vi "bus_button.vi"(3 "Container State":T3 caption="컨테이너 상태", 4 "Previous State":variant caption="이전 상태", 5 "Previous Version":T2 caption="이전 버전") -> (2 "Current State":T1 caption="현재 상태")   [LabVIEW 2014, in "bus_button.xctl"]
uses:
  bus_button.xctl
  Normal.ctl
  <vilib>/_xctls/Container State.ctl
  <vilib>/_xctls/Version.ctl
  <vilib>/_xctls/XControlSupport.lvlib
panel:
  in  "Default Indicator State":T1 caption="기본 인디케이터 상태"
  in  "Default Control State":T1 caption="기본 컨트롤 상태"
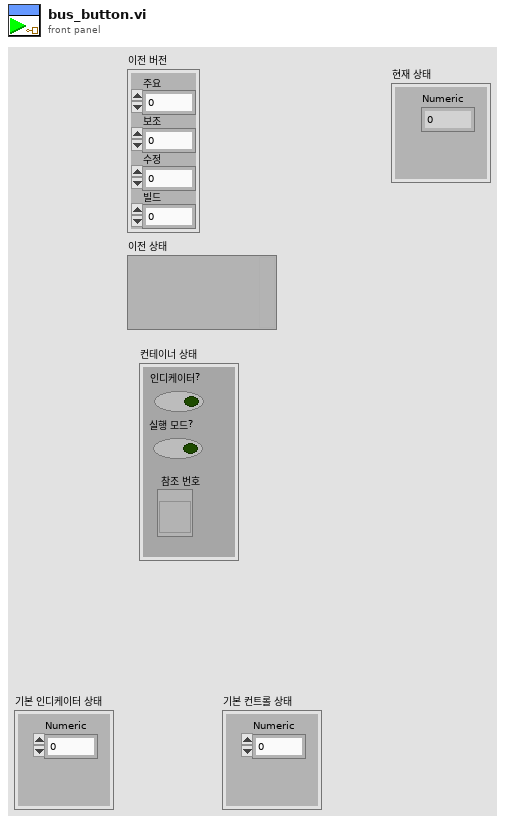
[diagram p1: front panel]
types:
  T1 = typedef "bus_button.xctl/Normal.ctl" = cluster{"Numeric":dbl}
  T2 = typedef "XControlSupport.lvlib/Version.ctl" = cluster{"Major":u16, "Minor":u16, "Fix":u16, "Build":u16}
  T3 = typedef "XControlSupport.lvlib/Container State.ctl" = cluster{"Indicator?":bool, "Run Mode?":bool, " Refnum":refnum<vi>}
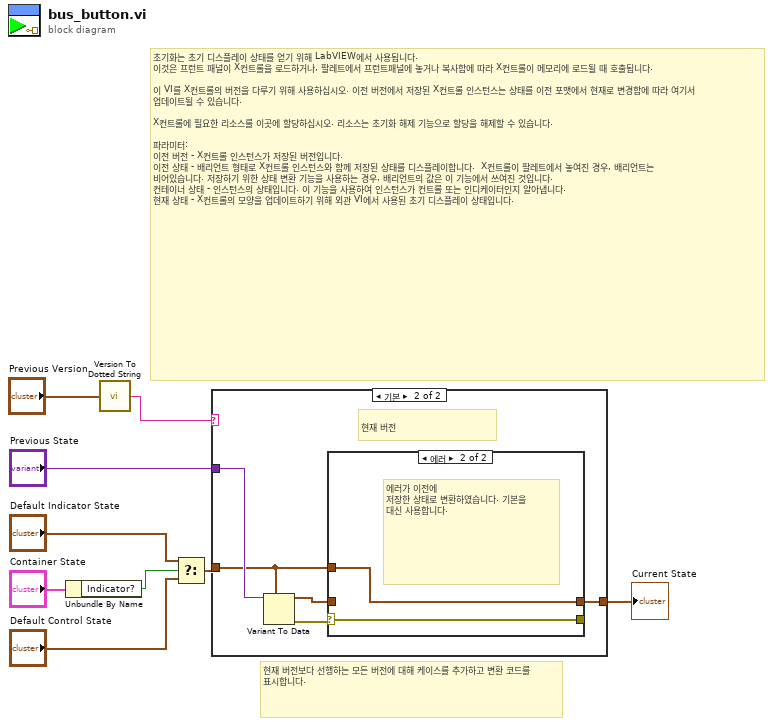
[diagram p0: block diagram]
diagram:
  # "현재 버전보다 선행하는 모든 버전에 대해 케이스를 추가하고 변환 코드를 표시합니다."
  # "초기화는 초기 디스플레이 상태를 얻기 위해 LabVIEW에서 사용됩니다.\n이것은 프런트 패널이 X컨트롤을 로드하거나, 팔레트에서 프런트패널에 놓거나 복사함에 따라 X컨트롤이 메모리에 로드될 때 호출됩니다.\n\n이 VI를 X컨트롤의 버전을 다루기 위해 사용하십시오. 이전 버전에서 저장된 X컨트롤 인스턴스는 상태를 이전 포맷에서 현재로 변경함에 따라 여기서 업데이트될 수 있습니다.\n\nX컨트롤에 필요한 리소스를 이곳에 할당하십시오. 리소스는 초기화 해제 기능으로 할당을 해제할 수 있습니다.\n\n파라미터:\n이전 버전 - X컨트롤 인스턴스가 저장된 버전입니다.\n이전 상태 - 배리언트 형태로 X컨트롤 인스턴스와 함께 저장된 상태를 디스플레이합니다.  X컨트롤이 팔레트에서 놓여진 경우, 배리언트는 비어있습니다. 저장하기 위한 상태 변환 기능을 사용하는 경우, 배리언트의 값은 이 기능에서 쓰여진 것입니다. \n컨테이너 상태 - 인스턴스의 상태입니다. 이 기능을 사용하여 인스턴스가 컨트롤 또는 인디케이터인지 알아냅니다.\n현재 상태 - X컨트롤의 모양을 업데이트하기 위해 외관 VI에서 사용된 초기 디스플레이 상태입니다."
  n1 = Unbundle By Name("Container State") -> ("Indicator?"=w4:bool)
  n2 = call <vilib>:"Version To Dotted String.vi"("Version"="Previous Version") -> ("String Version"=w1:string)
  n3 = Select(t="Default Indicator State", s=w4, f="Default Control State") -> (s? t:f=w3:T1)
  n4 = case shown="기본" w1 {
    tunnel: "Previous State" -> [_ w15]
    tunnel: [w10 w11] -> w8
    tunnel: w3 -> [w10 w12]
    frame "0.0.0.0" {
      # "방금 생성됨, 기본 상태 사용"
    }
    frame Default {
      # "현재 버전"
      n5 = Variant To Data(type=w12, Variant=w15) -> (data=w13:T1, error out=w14:errorcluster)  [unwired: 1 in]
      n6 = case shown="에러" w14 {
        selector: w14 -> [w17 w18]
        tunnel: w13 -> [w16 _]
        tunnel: [w16 w19] -> w11
        tunnel: w12 -> [_ w19]
        tunnel: [w17 w18] -> _
        frame No Error {
        }
        frame Error {
          # "에러가 이전에\n저장한 상태로 변환하였습니다. 기본을 대신 사용합니다."
        }
      }
    }
  }
  "Current State" <- w8
